vi "Destroy.vi"(0 "reference in":refnum<class "NI-DAQmx.lvclass">, 5 "error in (no error)":errorcluster) -> (14 "reference out":refnum<class "NI-DAQmx.lvclass">, 19 "error out":errorcluster)   [LabVIEW 2020, in "NI-DAQmx.lvclass"]
uses:
  NI-DAQmx.lvclass
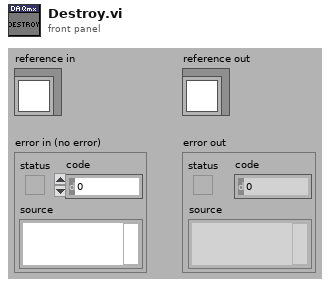
[diagram p1: front panel]
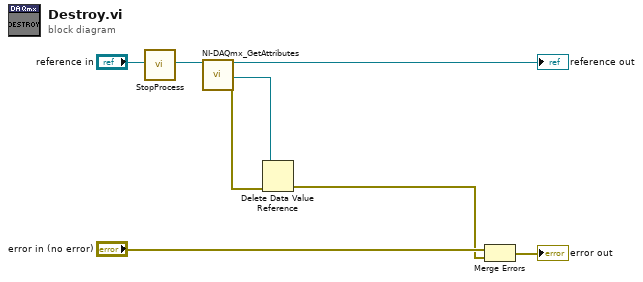
[diagram p0: block diagram]
diagram:
  n1 = call "StopProcess.vi"("reference in"="reference in") -> ("reference out"=w1:refnum<class "NI-DAQmx.lvclass">)  [unwired: 17 in, 1 out]
  n2 = call "NI-DAQmx_GetAttributes.vi"("reference in"=w1) -> ("reference out"=→"reference out":refnum<class "NI-DAQmx.lvclass">, "DataRef"=w5:refnum<data-value>, "error out"=w6:errorcluster)  [unwired: 15 in, 1 out]
  n3 = Delete Data Value Reference(data value reference=w5, error in=w6) -> (error out=w3:errorcluster)  [unwired: 1 out]
  n4 = Merge Errors("error in (no error)", w3) -> (→"error out":errorcluster)
